vi "Is in range.vi"(8 "error in (no error)":errorcluster, 9 "Deviation":refnum<class "Mag Lab Result.lvclass">, 10 "Center":refnum<class "Mag Lab Result.lvclass">, 11 "DBL Result in":refnum<class "DBL Result.lvclass">) -> (0 "error out":errorcluster, 3 "DBL Result out":refnum<class "DBL Result.lvclass">, 4 "Is in range?":bool)   [LabVIEW 2015, in "DBL Result.lvclass"]
uses:
  DBL Result.lvclass
  Mag Lab Result.lvclass
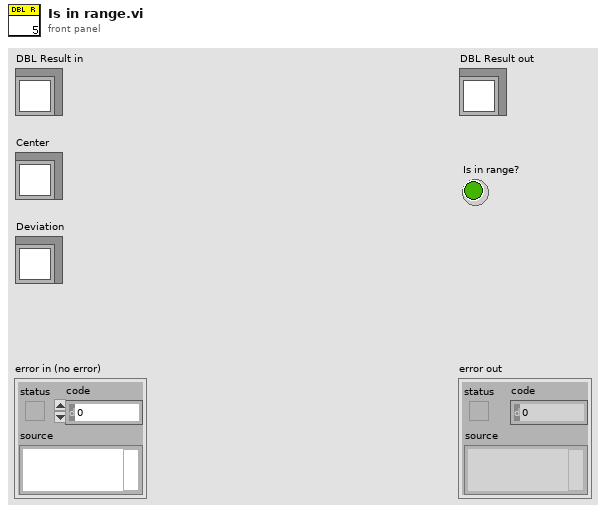
[diagram p1: front panel]
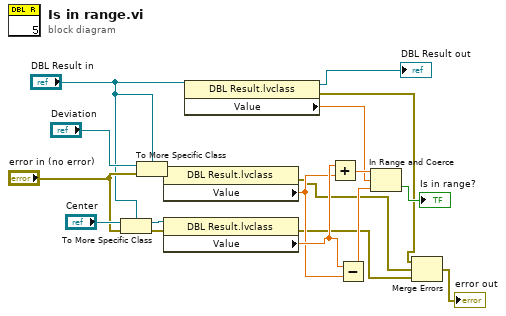
[diagram p0: block diagram]
diagram:
  n1 = To More Specific Class(target class="DBL Result in", reference="Center", error in="error in (no error)") -> (specific class reference=w14:refnum<class "DBL Result.lvclass">, error out=w15:errorcluster)
  n2 = To More Specific Class(target class="DBL Result in", reference="Deviation", error in="error in (no error)") -> (specific class reference=w13:refnum<class "DBL Result.lvclass">)  [unwired: 1 out]
  n3 = property class="DBL Result.lvclass"(reference=w13) -> (error out=w3:errorcluster, "Value"=w9:dbl)  [unwired: 1 in, 1 out]
  n4 = property class="DBL Result.lvclass"(reference=w14, error in=w15) -> (error out=w2:errorcluster, "Value"=w10:dbl)  [unwired: 1 out]
  n5 = property class="DBL Result.lvclass"(reference="DBL Result in") -> (reference out=→"DBL Result out":refnum<class "DBL Result.lvclass">, error out=w4:errorcluster, "Value"=w6:dbl)  [unwired: 1 in]
  n6 = Add(x=w10, y=w9) -> (x+y=w8:dbl)
  n7 = Subtract(x=w10, y=w9) -> (x-y=w7:dbl)
  n8 = In Range and Coerce(upper limit=w8, x=w6, lower limit=w7) -> (In Range?=→"Is in range?":bool)  [unwired: 1 out]
  n9 = Merge Errors(w4, w3, w2) -> (→"error out":errorcluster)
